vi "HEWH Temp Adjustment.vi"(0 "VISA session":refnum<visa-resource-name>="MW100", 2 "Semiphore":T1, 5 "Degrees Target(58)":dbl=3.0, 7 "Degrees reading":dbl, 9 "Degrees setting In":dbl=2.9360496277915633, 11 "Error In":errorcluster, 12 "Elapsed Time (sec)":dbl format="%.2f", 13 "Temp Adjust Time (3s)":dbl=3.0, 14 "K(0.1)":dbl=0.1) -> (4 "VISA session out":refnum<visa-resource-name>, 6 "Degree setting Out":dbl, 15 "Error Out":errorcluster)   [LabVIEW 2012]
uses:
  Intellifaucet/Intellfaucet Mode.ctl
panel:
  in  "ErrorPassBand(F)":dbl=1.0
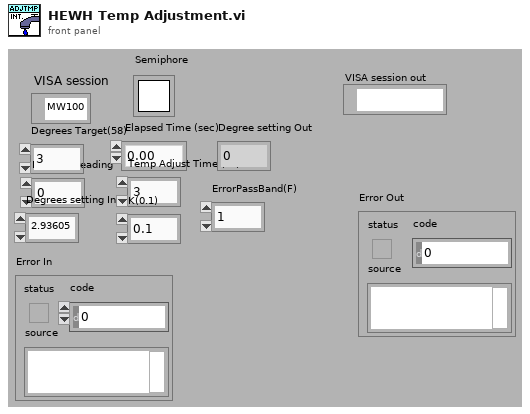
[diagram p1: front panel]
types:
  T1 = typedef "Semaphore RefNum" = refnum<k1>
  T2 = typedef "Intellfaucet Mode.ctl" = enum16{"Adjust Temp", "Adjust Flow", "Start Flow", "Stop Flow"}
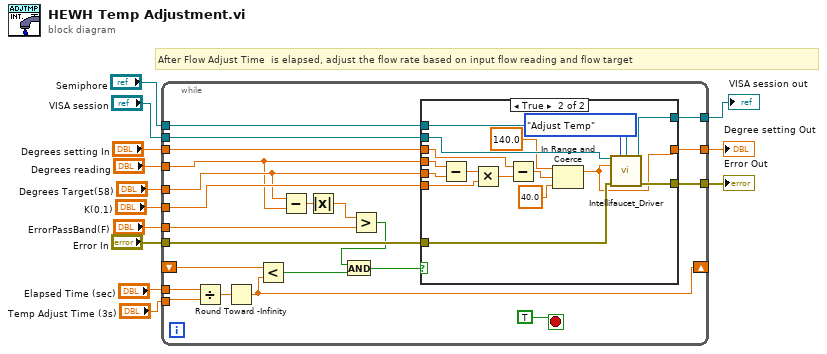
[diagram p0: block diagram]
diagram:
  # "After Flow Adjust Time  is elapsed, adjust the flow rate based on input flow reading and flow target"
  n1 = while {
    tunnel: "Elapsed Time (sec)" -> [w34]
    tunnel: "Temp Adjust Time (3s)" -> [w33]
    shift-right: [w23] -> _
    shift-left: _ -> [w24]
    tunnel: "VISA session" -> [w31]
    tunnel: "Semiphore" -> [w30]
    tunnel: "Error In" -> [w29]
    tunnel: [w28] -> w8
    tunnel: "Degrees reading" -> [w19]
    tunnel: "Degrees Target(58)" -> [w20]
    tunnel: "K(0.1)" -> [w27]
    tunnel: "Degrees setting In" -> [w26]
    tunnel: [w25] -> w3
    tunnel: [w22] -> w2
    tunnel: "ErrorPassBand(F)" -> [w16]
    stop <- TRUE stop-if-true
    n2 = Divide(x=w34, y=w33) -> (x/y=w32:dbl)
    n3 = Round Toward -Infinity(1:w32) -> (0:w23:dbl)
    n4 = Less?(x=w24, y=w23) -> (x < y?=w21:bool)
    n5 = Subtract(x=w20, y=w19) -> (x-y=w18:dbl)
    n6 = Absolute Value(x=w18) -> (abs(x)=w17:dbl)
    n7 = Greater?(x=w17, y=w16) -> (0:w15:bool)
    n8 = And(x=w15, y=w21) -> (x .and. y?=w14:bool)
    n9 = case shown="True" w14 {
      tunnel: w31 -> [w36 w53]
      tunnel: w30 -> [_ w52]
      tunnel: w29 -> [w38 w51]
      tunnel: [w38 w50] -> w28
      tunnel: w27 -> [_ w48]
      tunnel: w20 -> [_ w47]
      tunnel: w19 -> [_ w46]
      tunnel: w26 -> [w37 w44]
      tunnel: [w37 w39] -> w25
      tunnel: [w36 w43] -> w22
      frame False {
      }
      frame True {
        n10 = Subtract(x=w46, y=w47) -> (x-y=w49:dbl)
        n11 = Multiply(x=w49, y=w48) -> (x*y=w45:dbl)
        n12 = Subtract(x=w44, y=w45) -> (x-y=w42:dbl)
        n13 = In Range and Coerce(upper limit=140.0, x=w42, lower limit=40.0) -> (coerced(x)=w39:dbl)  [unwired: 1 out]
        n14 = call "Intellifaucet_Driver.vi"("VISA session"=w53, "Mode"=Intellfaucet_Mode."Adjust Temp", "Semiphore"=w52, "Temperature(F)"=w39, "Error In"=w51) -> ("VISA session out"=w43:refnum<visa-resource-name>, "Error Out"=w50:errorcluster)  [unwired: 9 in]
      }
    }
  }
  "Error Out" <- w8
  "Degree setting Out" <- w3
  "VISA session out" <- w2
